vi "FormCalibra9_motorAllON.vi"() -> ()   [LabVIEW 2014]
uses:
  testMachine.ctl
  mainMachine.ctl
  <vilib>/Analysis/baseanly.llb/Mean (DBL).vi
  <vilib>/express/express shared/transition.llb/Dynamic To Waveform Array.vi
  <vilib>/express/express signal manip/GetorSetDDTAttributes/Set DDT Attributes/SetT0.vi
  <vilib>/express/express shared/transition.llb/Waveform Array To Dynamic.vi
  <vilib>/measure/mamon.llb/Trigger Detection for 1 Channel.vi
  <vilib>/express/express signal manip/GetorSetDDTAttributes/Set DDT Attributes/Set DDT Properties.xnode
  <vilib>/Analysis/NI_AALBase.lvlib
  <resource>/objmgr/daqmx.rc
  <vilib>/measure/NI_MAPro.lvlib
panel:
  out "editDistance":dbl caption="Distancia (m)" format="%#_4f"
  in  "Lower level":dbl
  in  "hysteresis":dbl format="%.2p"
  in  "level":dbl format="%.2p"
  out "rpm":bool
  out "deviceName":tag
  out "editTotalWaitLimit":u8
  out "editCountWaitLimit":u8
  out "ledWaitState":bool caption="Wait State"
  out "sliderWaitUpperTime":u8(slide) max=50 scale=0.0..10.0
  out "slideWaitLowerTime":u8(slide) max=30 scale=0.0..1.0
  out "slideWaitTime":u8(slide) scale=0.0..1.0
  out "labelTestTime":string caption="Tempo total de ensaio"
  in  "buttonAcquisition":bool
  in  "editSetWaitTime":u8 caption="Tempo entre ciclos (s)" step=1 format="%0d"
  in  "stop":bool
  out "error out":errorcluster
  out "ledAcquireState":bool caption="Acquire State"
  out "editTotalLowerLimit":u8
  out "editCountLowerLimit":u8
  out "editTotalUpperLimit":u8
  out "editCountUpperLimit":u8
  out "ledEnsaio 3":bool
  out "ledBrakeState":bool caption="Brake State"
  out "ledExitState":bool caption="Exit State"
  out "ledMotorState":bool caption="Motor State"
  out "ledInit2State":bool caption="Init State"
  out "ledBlockState":bool caption="Block State"
  out "ledRunningState":bool caption="Running State"
  out "ledReadyState":bool caption="Ready State"
  out "ledInitState":bool caption="Init State"
  out "mainMachine":T1
  out "testMachine":T2=enum."finish"
  in  "editSetPathToFile":path
  in  "buttonStop":bool
  in  "buttonStart":bool
  out "graphForce":dynamicdata(graph)
  in  "editOffsetForce":dbl caption="Tara" min=0.0 max=100.0 step=0.1
  in  "editSetForce":dbl caption="Fator de conversão"
  out "editForce":dbl caption="Força (Kgf)" format="%#_4f"
  out "graphSpeed":dynamicdata(graph)
  in  "editSetSpeed":dbl caption="Fator de conversão"
  out "editSpeed":dbl caption="Velocidade (km/h)" format="%#_4f"
  out "editEngineSpeed":dbl caption="Rotação (RPM)" format="%#_4f"
  in  "buttonMotor":bool
  in  "buttonBrake":bool
  in  "editSetWaitLowerTime":u8 caption="Tempo de espera (s)"
  in  "editSetWaitUpperTime":u8=3 caption="Tempo de espera (s)"
  in  "editSetNumberOfCycles":u16 caption="Número de ciclos" max=999 step=1 format="%0d"
  in  "editSetLowerLimit":u32 caption="Limite inferior (km/h)"
  in  "editSetUpperLimit":u32 caption="Limite superior (km/h)"
  out "editTempB":dbl caption="Temperatura B (ºC)"
  out "editTempA":dbl caption="Temperatura A (ºC)"
  in  "editSetTempRef":dbl caption="Offset referência" step=0.01 format="%#_2f"
  out "editTempRef":dbl caption="Referência (ºC)"
  out "ledMotor":bool
  out "ledBrake":bool
  out "ledEnsaio":bool
  out "labelTotalCycle":string
  out "labelCurrentCycle":string
  out "labelSystemTitle":string
  in  "editCurrCycleCtr":u32
  in  "velocidade 2":u32
  out "velocidade":u32
  # "Bancada de Frenagem - Ensaio"
  # "Ensaio"
  # "Temperatura"
  # "Rotação"
  # "Célula de Carga"
  # "Configurações do ensaio"
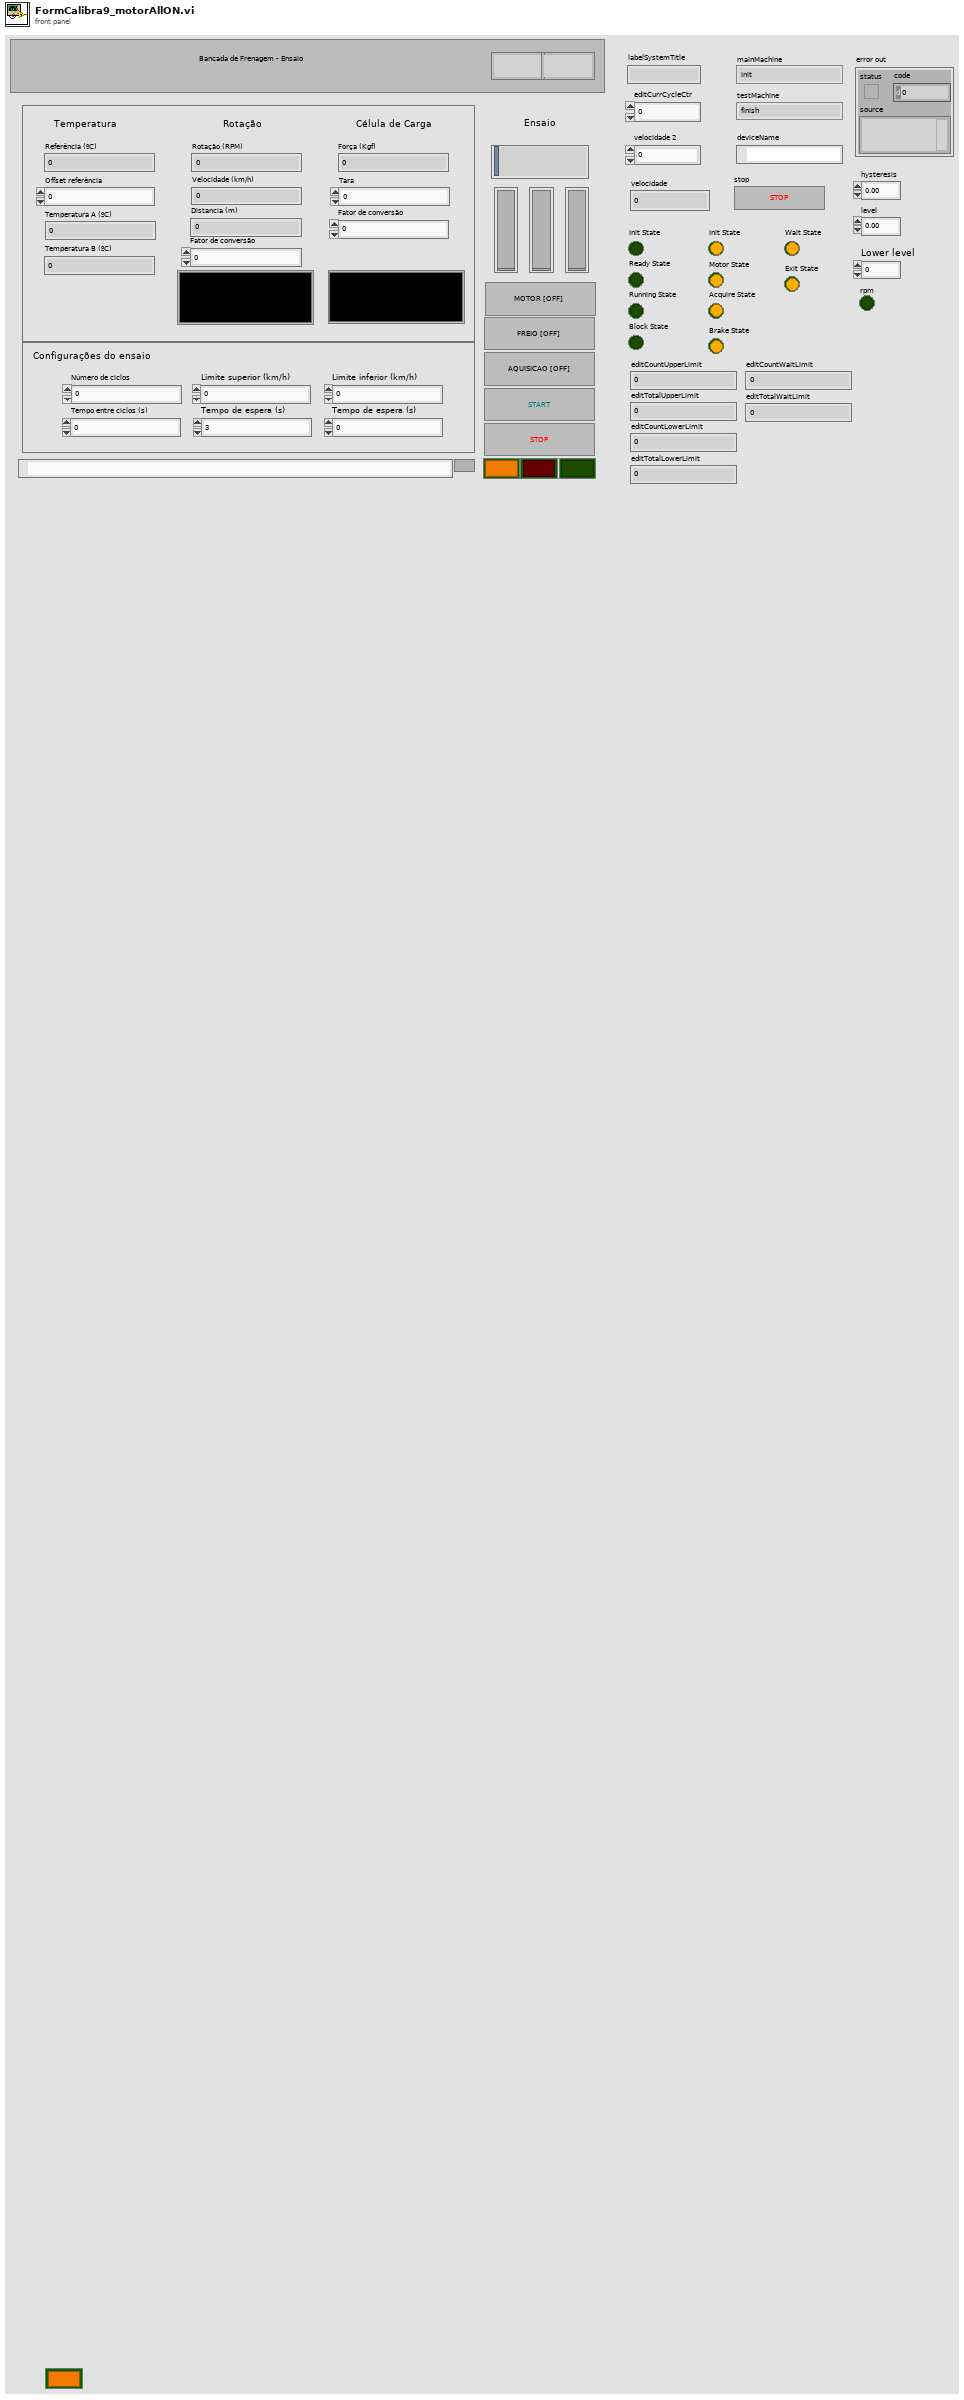
[diagram p1: front panel]
types:
  T1 = typedef "mainMachine.ctl" = enum16{"init", "ready", "running", "blocked", "finish"}
  T2 = typedef "testMachine.ctl" = enum16{"init", "motor", "motor acquire", "brake", "brake acquire", "wait ", "finish", "exit"}
  T3 = enum8{"Enabled", "Disabled", "Disabled and Grayed Out"}
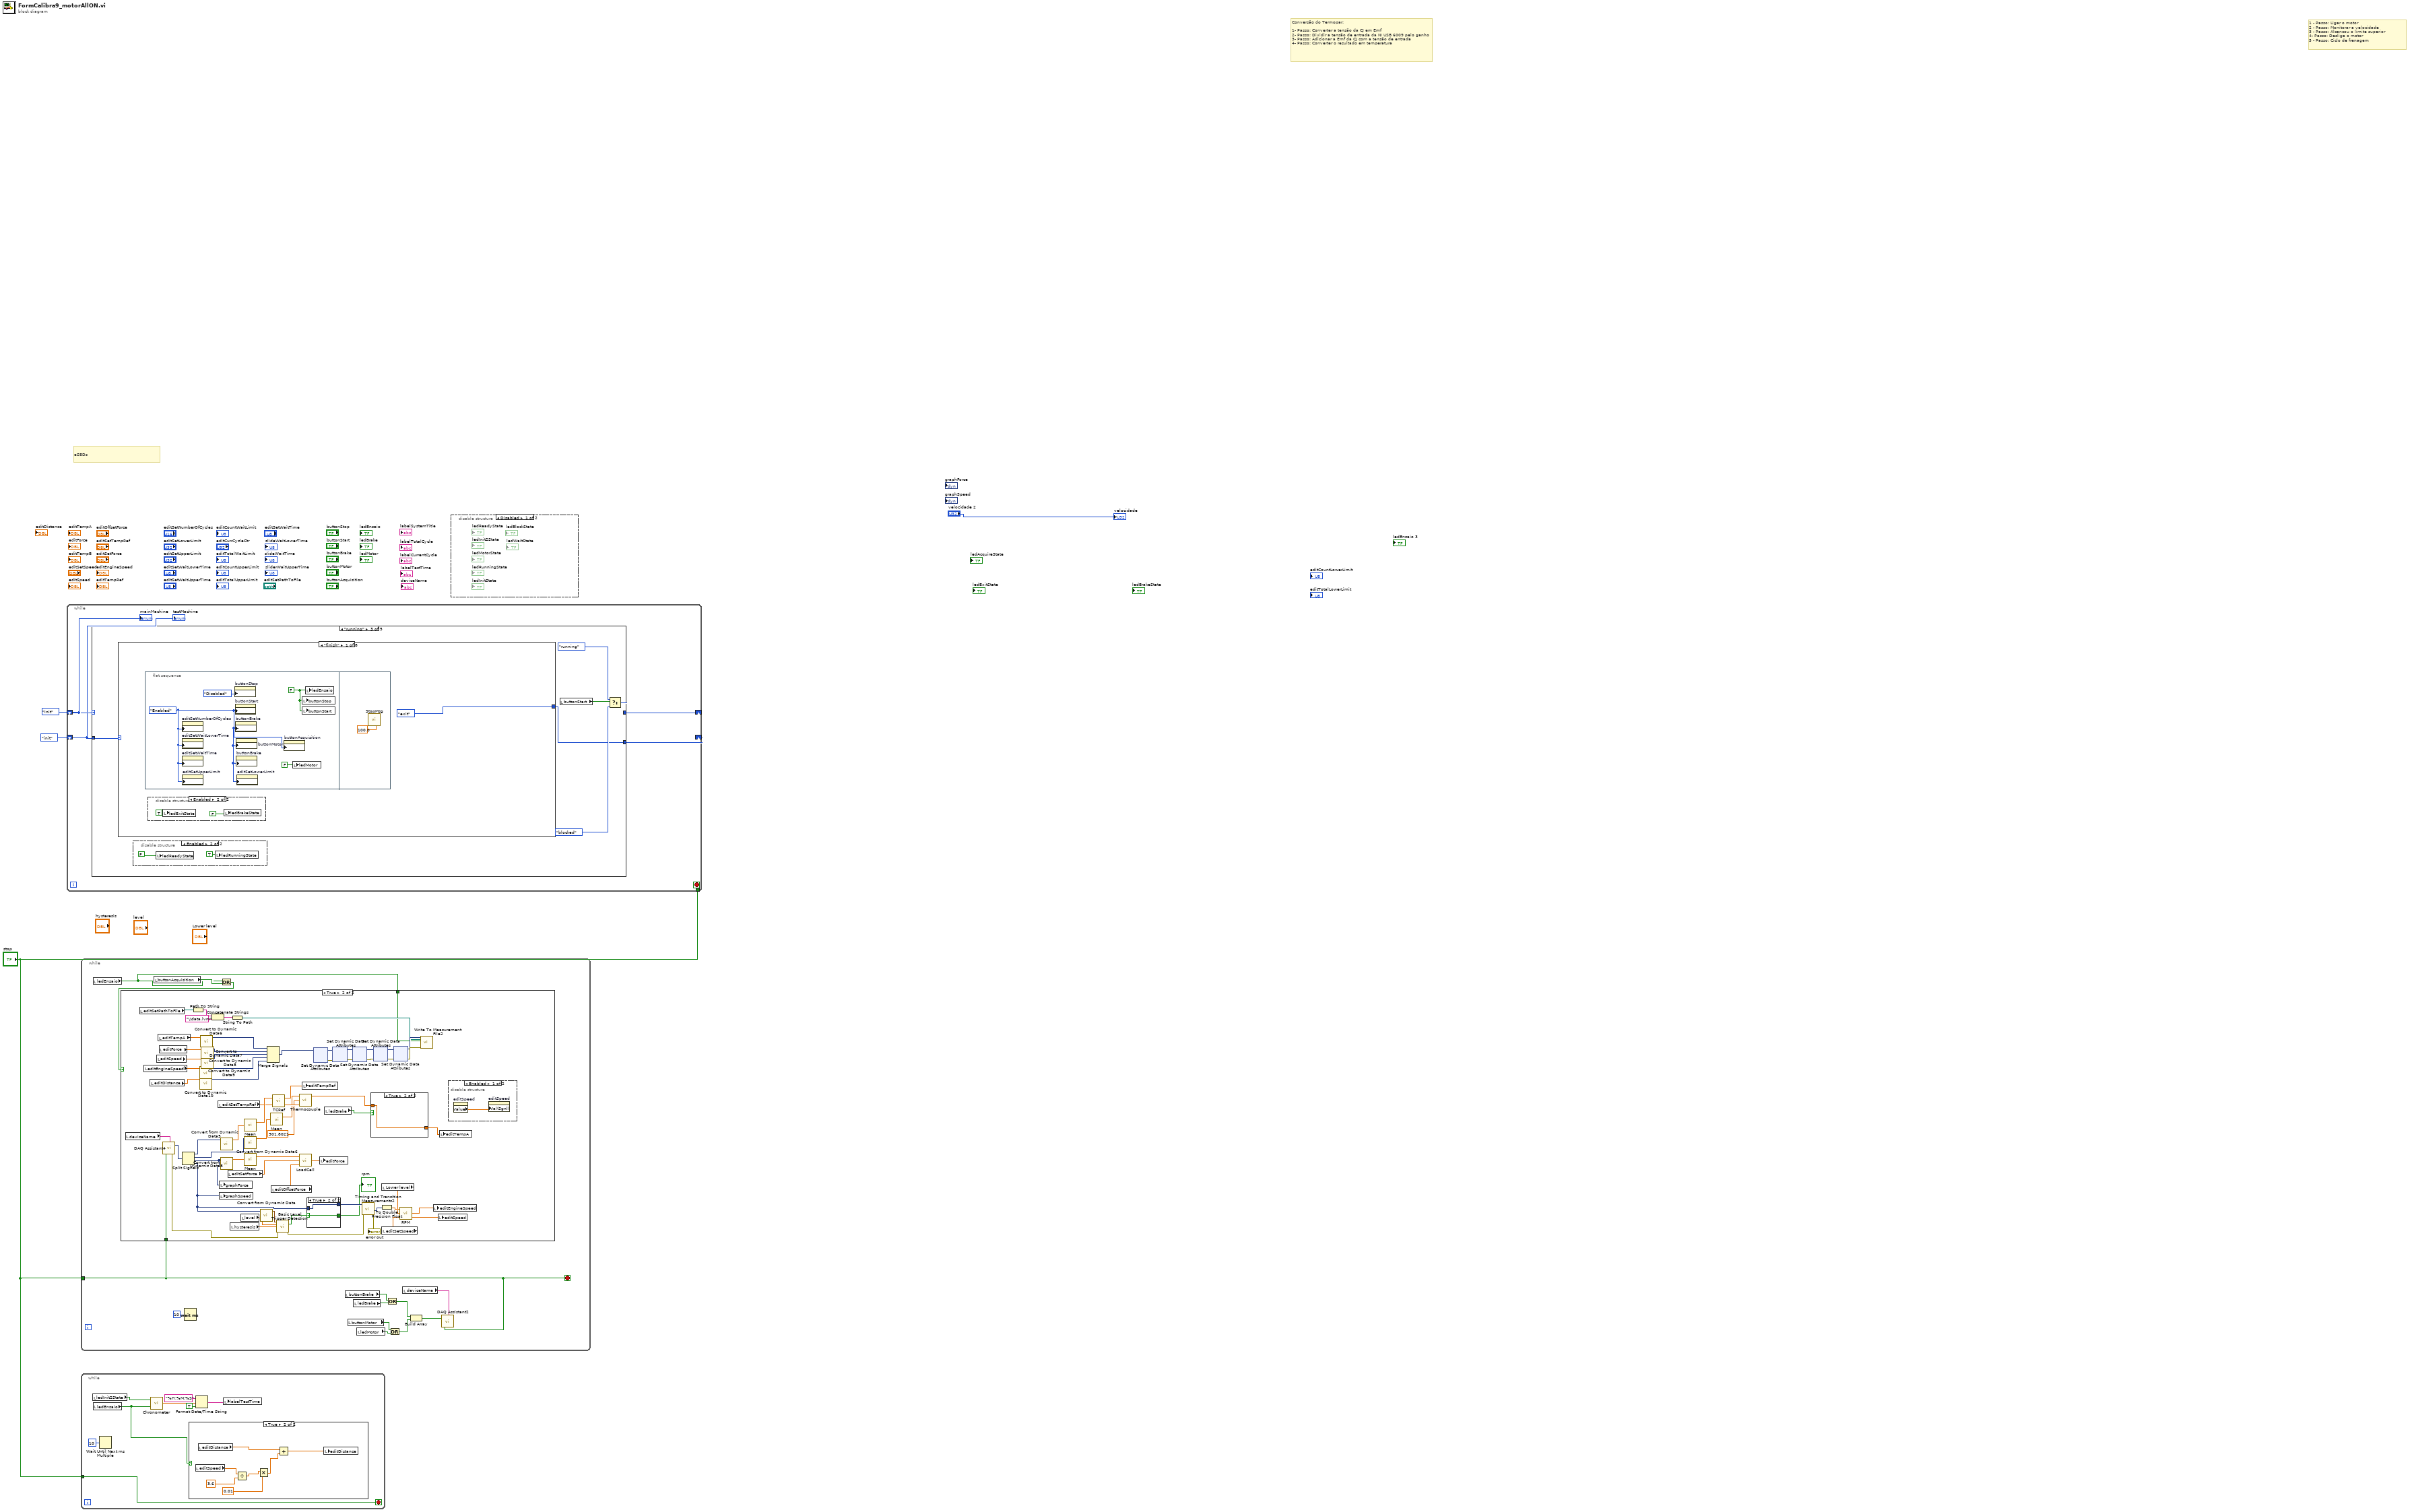
[diagram p0: block diagram]
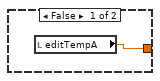
[diagram p5: hidden frame]
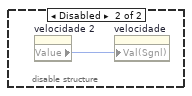
[diagram p7: hidden frame]
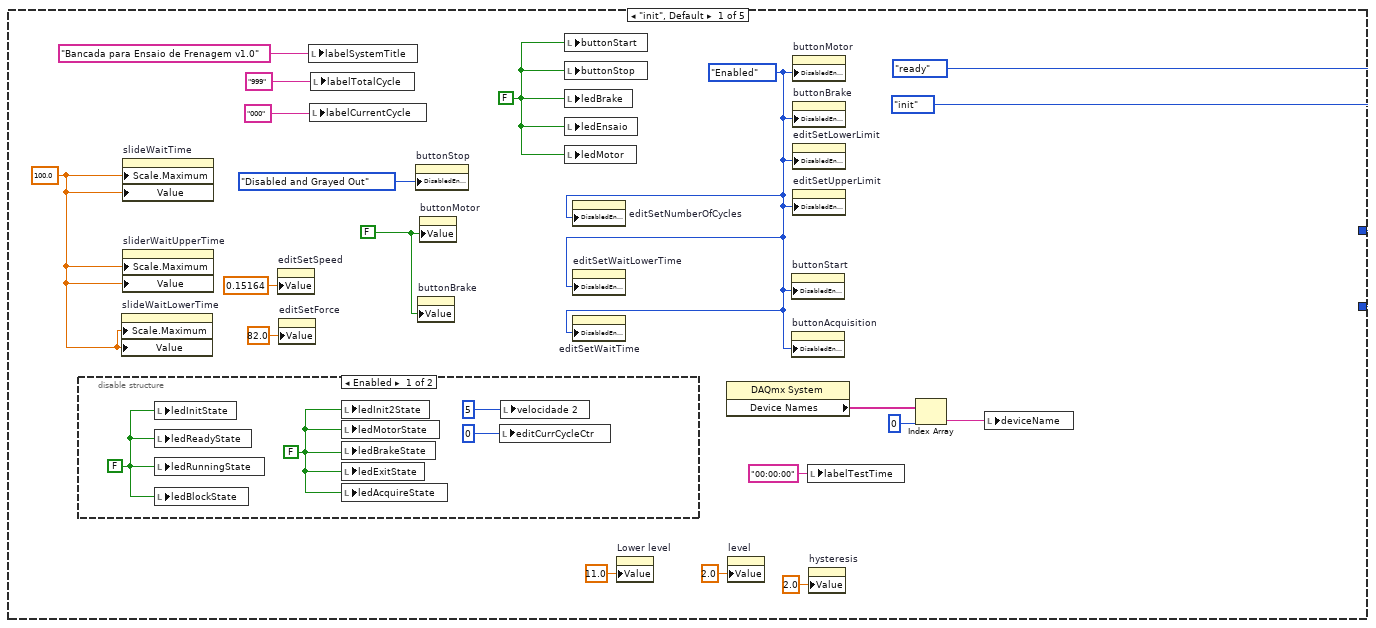
[diagram p8: hidden frame]
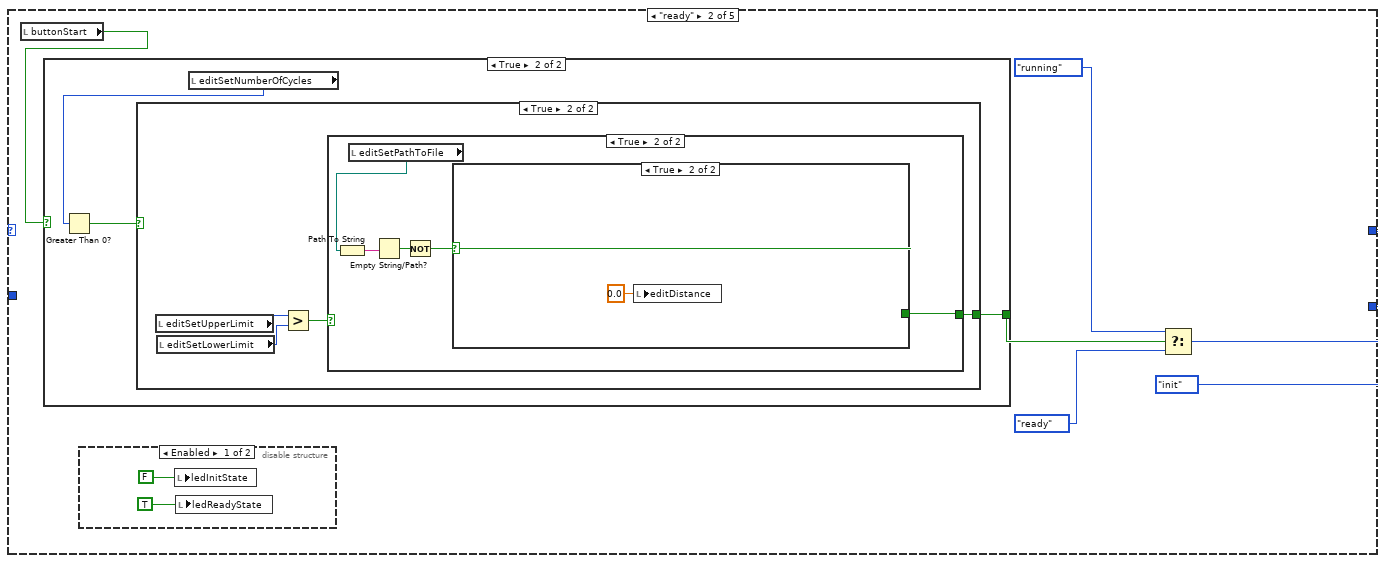
[diagram p10: hidden frame]
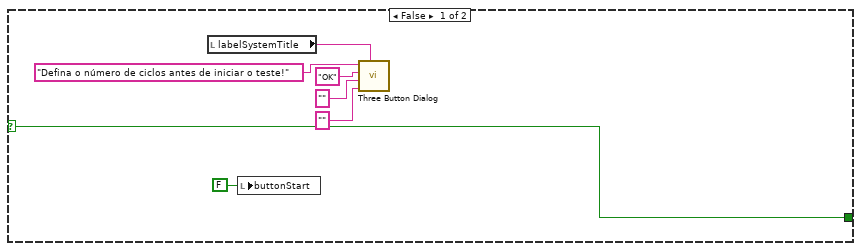
[diagram p13: hidden frame]
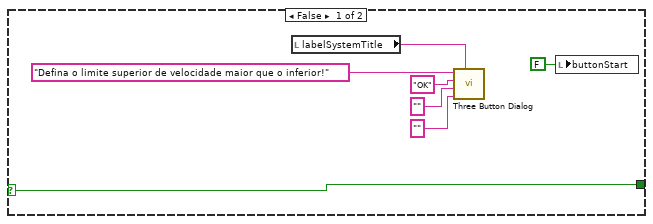
[diagram p14: hidden frame]
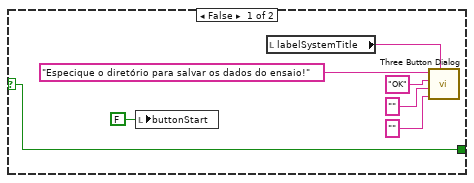
[diagram p15: hidden frame]
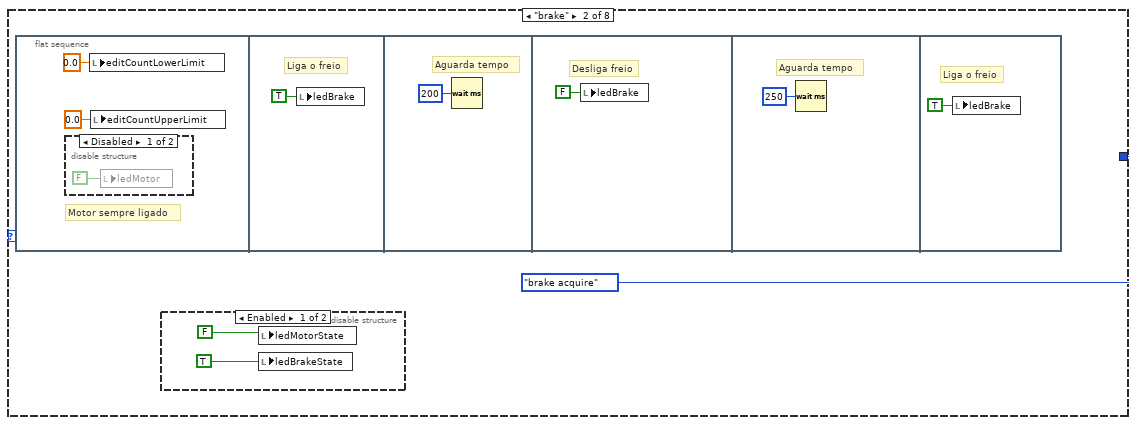
[diagram p18: hidden frame]
diagram:
  # "eSEDs"
  # "1 - Passo: Ligar o motor\n2 - Passo: Monitorar a velocidade\n3 - Passo: Alcancou o limite superior\n4- Passo: Desliga o motor\n5 - Passo: Ciclo de frenagem"
  # "Conversão do Termopar:\n\n1- Passo: Converter a tensão da CJ em Emf\n2- Passo: Dividir a tensão de entrada da NI USB 6009 pelo ganho\n3- Passo: Adicionar a Emf da CJ com a tensão de entrada\n4- Passo: Converter o resultado em temperatura"
  n1 = while {
    shift-right: [w9] -> _
    shift-left: mainMachine."init" ("mainMachine") -> [w6]
    shift-right: [w8] -> _
    shift-left: testMachine."init" ("testMachine") -> [w7]
    tunnel: "stop" -> [w5]
    stop <- w5 stop-if-true
    n2 = case shown="\"running\"" w6 {
      tunnel: [mainMachine."ready" ("mainMachine") w33 w79 w224 mainMachine."finish" ("mainMachine")] -> w9
      tunnel: [testMachine."init" ("testMachine") testMachine."init" ("testMachine") w78 testMachine."init" ("testMachine") testMachine."init" ("testMachine")] -> w8
      tunnel: w7 -> [_ _ w77 _ _]
      frame "init", Default {
        w19 = 100.0 ("Scale.Range:Maximum")
        w20 = T3."Enabled" ("Disabled")
        w21 = FALSE ("buttonMotor")
        w27 = FALSE ("motor")
        n3 = disable-structure shown="Enabled" {
          frame Enabled {
            w29 = FALSE
            w30 = FALSE
            n4 = local write "ledInitState"(w30) -> ()
            n5 = local write "ledReadyState"(w30) -> ()
            n6 = local write "ledRunningState"(w30) -> ()
            n7 = local write "ledBlockState"(w30) -> ()
            n8 = local write "ledInit2State"(w29) -> ()
            n9 = local write "ledMotorState"(w29) -> ()
            n10 = local write "ledBrakeState"(w29) -> ()
            n11 = local write "ledExitState"(w29) -> ()
            n12 = local write "ledAcquireState"(w29) -> ()
            n13 = local write "editCurrCycleCtr"(u32 0 ("currentCycleCtr")) -> ()
            n14 = local write "velocidade 2"(u32 5 ("velocidade 2")) -> ()
          }
          frame Disabled {
          }
        }
        n15 = property on="slideWaitLowerTime" class="Slide (strict)"("Scale.Maximum"=w19, "Value"=w19) -> ()  [unwired: 2 in, 2 out]
        n16 = property on="slideWaitTime" class="Slide (strict)"("Scale.Maximum"=w19, "Value"=w19) -> ()  [unwired: 2 in, 2 out]
        n17 = property on="sliderWaitUpperTime" class="Slide (strict)"("Scale.Maximum"=w19, "Value"=w19) -> ()  [unwired: 2 in, 2 out]
        n18 = property on="editSetSpeed" class="DigNum (strict)"("Value"=0.15164 ("editSetSpeed")) -> ()  [unwired: 2 in, 2 out]
        n19 = property on="editSetForce" class="DigNum (strict)"("Value"=82.0 ("editSetForce")) -> ()  [unwired: 2 in, 2 out]
        n20 = local write "labelSystemTitle"("Bancada para Ensaio de Frenagem v1.0" ("systemTitle")) -> ()
        n21 = local write "labelCurrentCycle"("000" ("currentCycle")) -> ()
        n22 = local write "labelTotalCycle"("999" ("totalCycle")) -> ()
        n23 = property on="buttonStop" class="Bool (strict)"("DisabledEnum"=T3."Disabled and Grayed Out" ("Disabled")) -> ()  [unwired: 2 in, 2 out]
        n24 = property on="buttonBrake" class="Bool (strict)"("Value"=w21) -> ()  [unwired: 2 in, 2 out]
        n25 = property on="buttonMotor" class="Bool (strict)"("Value"=w21) -> ()  [unwired: 2 in, 2 out]
        n26 = local write "buttonStart"(w27) -> ()
        n27 = local write "buttonStop"(w27) -> ()
        n28 = local write "ledBrake"(w27) -> ()
        n29 = local write "ledEnsaio"(w27) -> ()
        n30 = local write "ledMotor"(w27) -> ()
        n31 = property on="editSetNumberOfCycles" class="DigNum (strict)"("DisabledEnum"=w20) -> ()  [unwired: 2 in, 2 out]
        n32 = property on="editSetWaitLowerTime" class="DigNum (strict)"("DisabledEnum"=w20) -> ()  [unwired: 2 in, 2 out]
        n33 = property on="editSetWaitTime" class="DigNum (strict)"("DisabledEnum"=w20) -> ()  [unwired: 2 in, 2 out]
        n34 = property on="Lower level" class="DigNum (strict)"("Value"=11.0 ("Lower level")) -> ()  [unwired: 2 in, 2 out]
        n35 = property class="DAQmx System"() -> ("Device Names"=w18:tag[])  [unwired: 2 in, 2 out]
        n36 = property on="level" class="DigNum (strict)"("Value"=2.0 ("level")) -> ()  [unwired: 2 in, 2 out]
        n37 = property on="buttonStart" class="Bool (strict)"("DisabledEnum"=w20) -> ()  [unwired: 2 in, 2 out]
        n38 = property on="buttonAcquisition" class="Bool (strict)"("DisabledEnum"=w20) -> ()  [unwired: 2 in, 2 out]
        n39 = property on="buttonMotor" class="Bool (strict)"("DisabledEnum"=w20) -> ()  [unwired: 2 in, 2 out]
        n40 = property on="buttonBrake" class="Bool (strict)"("DisabledEnum"=w20) -> ()  [unwired: 2 in, 2 out]
        n41 = property on="editSetLowerLimit" class="DigNum (strict)"("DisabledEnum"=w20) -> ()  [unwired: 2 in, 2 out]
        n42 = property on="editSetUpperLimit" class="DigNum (strict)"("DisabledEnum"=w20) -> ()  [unwired: 2 in, 2 out]
        n43 = local write "labelTestTime"("00:00:00" ("labelTestTime")) -> ()
        n44 = property on="hysteresis" class="DigNum (strict)"("Value"=2.0 ("hysteresis")) -> ()  [unwired: 2 in, 2 out]
        n45 = Index Array(array=w18, index=0) -> (element=w16:tag)
        n46 = local write "deviceName"(w16) -> ()
      }
      frame "ready" {
        n47 = local read "buttonStart"() -> (w36:bool)
        n48 = case shown="True" w36 {
          selector: w36 -> [w41 _]
          tunnel: [w41 w42] -> w35
          frame False {
          }
          frame True {
            n49 = local read "editSetNumberOfCycles"() -> (w43:u16)
            n50 = Greater Than 0?(x=w43) -> (x > 0?=w44:bool)
            n51 = case shown="True" w44 {
              selector: w44 -> [w51 _]
              tunnel: [w51 w52] -> w42
              frame False {
                n52 = local read "labelSystemTitle"() -> (w46:string)
                n53 = local write "buttonStart"(FALSE ("startButton")) -> ()
                n54 = call <vilib>:"Three Button Dialog.vi"("Window Title (\"\")"=w46, "Right Button Text (\"Cancel\")"="" ("Right Button Text (\"Cancel\")"), "Center Button Text (\"No\")"="" ("Center Button Text (\"No\")"), "Left Button Text (\"Yes\")"="OK" ("Left Button Text (\"Yes\")"), "message"="Defina o número de ciclos antes de iniciar o teste!") -> ()  [unwired: 6 in, 1 out]
              }
              frame True {
                n55 = local read "editSetUpperLimit"() -> (w54:u32)
                n56 = local read "editSetLowerLimit"() -> (w53:u32)
                n57 = Greater?(x=w54, y=w53) -> (0:w55:bool)
                n58 = case shown="True" w55 {
                  selector: w55 -> [w62 _]
                  tunnel: [w62 w65] -> w52
                  frame False {
                    n59 = local read "labelSystemTitle"() -> (w57:string)
                    n60 = call <vilib>:"Three Button Dialog.vi"("Window Title (\"\")"=w57, "Right Button Text (\"Cancel\")"="" ("Right Button Text (\"Cancel\")"), "Center Button Text (\"No\")"="" ("Center Button Text (\"No\")"), "Left Button Text (\"Yes\")"="OK" ("Left Button Text (\"Yes\")"), "message"="Defina o limite superior de velocidade maior que o inferior!") -> ()  [unwired: 6 in, 1 out]
                    n61 = local write "buttonStart"(FALSE ("startButton")) -> ()
                  }
                  frame True {
                    n62 = local read "editSetPathToFile"() -> (w67:path)
                    n63 = Path To String(path=w67) -> (string=w66:string)
                    n64 = Empty String/Path?(string/path=w66) -> (empty?=w64:bool)
                    n65 = Not(x=w64) -> (.not. x?=w63:bool)
                    n66 = case shown="True" w63 {
                      selector: w63 -> [w74 w76]
                      tunnel: [w74 w76] -> w65
                      frame False {
                        n67 = local write "buttonStart"(FALSE ("startButton")) -> ()
                        n68 = local read "labelSystemTitle"() -> (w69:string)
                        n69 = call <vilib>:"Three Button Dialog.vi"("Window Title (\"\")"=w69, "Right Button Text (\"Cancel\")"="" ("Right Button Text (\"Cancel\")"), "Center Button Text (\"No\")"="" ("Center Button Text (\"No\")"), "Left Button Text (\"Yes\")"="OK" ("Left Button Text (\"Yes\")"), "message"="Especique o diretório para salvar os dados do ensaio!") -> ()  [unwired: 6 in, 1 out]
                      }
                      frame True {
                        n70 = local write "editDistance"(0.0 ("editDistance")) -> ()
                      }
                    }
                  }
                }
              }
            }
          }
        }
        n71 = disable-structure shown="Enabled" {
          frame Enabled {
            n72 = local write "ledInitState"(FALSE ("ledReady")) -> ()
            n73 = local write "ledReadyState"(TRUE ("ledReady")) -> ()
          }
          frame Disabled {
          }
        }
        n74 = Select(t=mainMachine."running" ("mainMachine"), s=w35, f=mainMachine."ready" ("mainMachine")) -> (s? t:f=w33:T1)
      }
      frame "running" {
        n75 = case shown="\"finish\"" w77 {
          tunnel: [testMachine."exit" ("testMachine") testMachine."brake acquire" ("testMachine") testMachine."motor acquire" ("testMachine") testMachine."motor" ("testMachine") w154 w174 testMachine."exit" ("testMachine") w207] -> w78
          frame "finish" {
            n76 = flat-sequence {
              frame #0 {
                w90 = FALSE ("ledReady")
                w89 = T3."Enabled" ("Disabled")
                n77 = property on="editSetNumberOfCycles" class="DigNum (strict)"("DisabledEnum"=w89) -> ()  [unwired: 2 in, 2 out]
                n78 = property on="editSetWaitLowerTime" class="DigNum (strict)"("DisabledEnum"=w89) -> ()  [unwired: 2 in, 2 out]
                n79 = property on="editSetWaitTime" class="DigNum (strict)"("DisabledEnum"=w89) -> ()  [unwired: 2 in, 2 out]
                n80 = property on="editSetUpperLimit" class="DigNum (strict)"("DisabledEnum"=w89) -> ()  [unwired: 2 in, 2 out]
                n81 = property on="buttonStop" class="Bool (strict)"("DisabledEnum"=T3."Disabled" ("Disabled")) -> ()  [unwired: 2 in, 2 out]
                n82 = property on="buttonStart" class="Bool (strict)"("DisabledEnum"=w89) -> ()  [unwired: 2 in, 2 out]
                n83 = property on="buttonBrake" class="Bool (strict)"("DisabledEnum"=w89) -> ()  [unwired: 2 in, 2 out]
                n84 = property on="buttonMotor" class="Bool (strict)"("DisabledEnum"=w89) -> ()  [unwired: 2 in, 2 out]
                n85 = property on="buttonBrake" class="Bool (strict)"("DisabledEnum"=w89) -> ()  [unwired: 2 in, 2 out]
                n86 = property on="editSetLowerLimit" class="DigNum (strict)"("DisabledEnum"=w89) -> ()  [unwired: 2 in, 2 out]
                n87 = property on="buttonAcquisition" class="Bool (strict)"("DisabledEnum"=w89) -> ()  [unwired: 2 in, 2 out]
                n88 = local write "ledMotor"(FALSE ("motor")) -> ()
                n89 = local write "buttonStop"(w90) -> ()
                n90 = local write "buttonStart"(w90) -> ()
                n91 = local write "ledEnsaio"(w90) -> ()
              }
              frame #1 {
                n92 = call "StopMsg.vi"("Max Value (100)"=100.0) -> ()  [unwired: 8 in, 2 out]
              }
            }
            n93 = disable-structure shown="Enabled" {
              frame Disabled {
              }
              frame Enabled {
                n94 = local write "ledExitState"(TRUE ("ledReady")) -> ()
                n95 = local write "ledBrakeState"(FALSE ("ledReady")) -> ()
              }
            }
          }
          frame "brake" {
            n96 = flat-sequence {
              frame #0 {
                # "Motor sempre ligado"
                n97 = disable-structure shown="Disabled" {
                  frame Disabled {
                    n98 = local write "ledMotor"(FALSE ("motor")) -> ()
                  }
                  frame Enabled {
                  }
                }
                n99 = local write "editCountLowerLimit"(0.0 ("editCountUpperLimit")) -> ()
                n100 = local write "editCountUpperLimit"(0.0 ("editCountUpperLimit")) -> ()
              }
              frame #1 {
                # "Liga o freio"
                n101 = local write "ledBrake"(TRUE ("freio")) -> ()
              }
              frame #2 {
                # "Aguarda tempo"
                n102 = Wait (ms)(milliseconds to wait=u32 200) -> ()  [unwired: 1 out]
              }
              frame #3 {
                # "Desliga freio"
                n103 = local write "ledBrake"(FALSE ("freio")) -> ()
              }
              frame #4 {
                # "Aguarda tempo"
                n104 = Wait (ms)(milliseconds to wait=u32 250) -> ()  [unwired: 1 out]
              }
              frame #5 {
                # "Liga o freio"
                n105 = local write "ledBrake"(TRUE ("freio")) -> ()
              }
            }
            n106 = disable-structure shown="Enabled" {
              frame Enabled {
                n107 = local write "ledMotorState"(FALSE ("ledReady")) -> ()
                n108 = local write "ledBrakeState"(TRUE ("ledReady")) -> ()
              }
              frame Disabled {
              }
            }
          }
          frame "motor" {
            n109 = flat-sequence {
              frame #0 {
                n110 = local read "editCurrCycleCtr"() -> (w109:u32)
                n111 = Increment(x=w109) -> (x+1=w108:u32)
                n112 = local write "editCurrCycleCtr"(w108) -> ()
              }
              frame #1 {
                n113 = local read "editCurrCycleCtr"() -> (w116:u32)
                n114 = local read "editTotalWaitLimit"() -> (w110:u8)
                n115 = local read "editTotalUpperLimit"() -> (w112:u8)
                n116 = local read "editTotalLowerLimit"() -> (w111:u8)
                n117 = local write "editCountLowerLimit"(u8 0 ("editCountLowerLimit")) -> ()
                n118 = local write "editCountWaitLimit"(u8 0 ("editCountWaitLimit")) -> ()
                n119 = local write "editCountUpperLimit"(u8 0 ("editCountUpperLimit")) -> ()
                n120 = Format Into String(format string="%03d", w116) -> (resulting string=w117:string)  [unwired: 2 in, 1 out]
                n121 = property on="sliderWaitUpperTime" class="Slide (strict)"("Value"=w112) -> ()  [unwired: 2 in, 2 out]
                n122 = property on="slideWaitLowerTime" class="Slide (strict)"("Value"=w111) -> ()  [unwired: 2 in, 2 out]
                n123 = property on="slideWaitTime" class="Slide (strict)"("Value"=w110) -> ()  [unwired: 2 in, 2 out]
                n124 = local write "labelCurrentCycle"(w117) -> ()
              }
              frame #2 {
                # "- Liga o motor"
                n125 = local write "ledMotor"(TRUE ("motor")) -> ()
                n126 = property on="buttonStop" class="Bool (strict)"("DisabledEnum"=T3."Enabled" ("Disabled")) -> ()  [unwired: 2 in, 2 out]
                n127 = property on="buttonStart" class="Bool (strict)"("DisabledEnum"=T3."Disabled and Grayed Out" ("Disabled")) -> ()  [unwired: 2 in, 2 out]
              }
            }
            n128 = disable-structure shown="Enabled" {
              frame Enabled {
                n129 = local write "ledInit2State"(FALSE ("ledReady")) -> ()
                n130 = local write "ledBrakeState"(FALSE ("ledReady")) -> ()
                n131 = local write "ledMotorState"(TRUE ("ledReady")) -> ()
              }
              frame Disabled {
              }
            }
          }
          frame "init", Default {
            n132 = stacked-sequence {
              frame #0 {
                w129 = FALSE ("ensaio")
                n133 = property on="buttonBrake" class="Bool (strict)"("Value"=w129) -> ()  [unwired: 2 in, 2 out]
                n134 = local write "ledMotor"(w129) -> ()
                n135 = local write "ledBrake"(w129) -> ()
                n136 = property on="buttonMotor" class="Bool (strict)"("Value"=w129) -> ()  [unwired: 2 in, 2 out]
                n137 = local read "editSetNumberOfCycles"() -> (w136:u16)
                n138 = local read "editSetWaitLowerTime"() -> (w130:u8)
                n139 = local read "editSetWaitUpperTime"() -> (w133:u8)
                n140 = local read "editSetWaitTime"() -> (w124:u8)
                n141 = Multiply(x=w124, y=u32 10) -> (x*y=w125:u32)
                n142 = Multiply(x=w130, y=u32 10) -> (x*y=w128:u32)
                n143 = Format Into String(format string="%03d", w136) -> (resulting string=w137:string)  [unwired: 2 in, 1 out]
                n144 = Multiply(x=w133, y=u32 10) -> (x*y=w127:u32)
                n145 = local write "editTotalLowerLimit"(w128) -> ()
                n146 = local write "editTotalUpperLimit"(w127) -> ()
                n147 = local write "editTotalWaitLimit"(w125) -> ()
                n148 = local write "labelTotalCycle"(w137) -> ()
                n149 = local write "editCurrCycleCtr"(u32 0 ("currentCycleCtr")) -> ()
                n150 = local write "labelCurrentCycle"("000" ("currentCycle")) -> ()
              }
              frame #1 {
                w145 = T3."Disabled" ("Disabled")
                n151 = property on="editSetNumberOfCycles" class="DigNum (strict)"("DisabledEnum"=w145) -> ()  [unwired: 2 in, 2 out]
                n152 = property on="editSetWaitLowerTime" class="DigNum (strict)"("DisabledEnum"=w145) -> ()  [unwired: 2 in, 2 out]
                n153 = property on="editSetWaitTime" class="DigNum (strict)"("DisabledEnum"=w145) -> ()  [unwired: 2 in, 2 out]
                n154 = local read "editTotalUpperLimit"() -> (w148:u8)
                n155 = property on="sliderWaitUpperTime" class="Slide (strict)"("Scale.Maximum"=w148, "Scale.Minimum"=0.0 ("Scale.Range:Minimum"), "Scale.Increment"=1.0 ("Scale.Range:Increment"), "Value"=w148) -> ()  [unwired: 2 in, 2 out]
                n156 = property on="buttonAcquisition" class="Bool (strict)"("DisabledEnum"=w145) -> ()  [unwired: 2 in, 2 out]
                n157 = local read "editTotalLowerLimit"() -> (w142:u8)
                n158 = property on="slideWaitLowerTime" class="Slide (strict)"("Scale.Maximum"=w142, "Scale.Minimum"=0.0 ("Scale.Range:Minimum"), "Scale.Increment"=1.0 ("Scale.Range:Increment"), "Value"=w142) -> ()  [unwired: 2 in, 2 out]
                n159 = local read "editTotalWaitLimit"() -> (w139:u8)
                n160 = property on="slideWaitTime" class="Slide (strict)"("Scale.Maximum"=w139, "Scale.Minimum"=0.0 ("Scale.Range:Minimum"), "Scale.Increment"=1.0 ("Scale.Range:Increment"), "Value"=w139) -> ()  [unwired: 2 in, 2 out]
                n161 = call "StarMsg.vi"("Show"=TRUE, "Max Value (100)"=100.0) -> ()  [unwired: 7 in, 2 out]
                n162 = property on="buttonMotor" class="Bool (strict)"("DisabledEnum"=w145) -> ()  [unwired: 2 in, 2 out]
                n163 = property on="buttonBrake" class="Bool (strict)"("DisabledEnum"=w145) -> ()  [unwired: 2 in, 2 out]
                n164 = property on="editSetLowerLimit" class="DigNum (strict)"("DisabledEnum"=w145) -> ()  [unwired: 2 in, 2 out]
                n165 = property on="editSetUpperLimit" class="DigNum (strict)"("DisabledEnum"=w145) -> ()  [unwired: 2 in, 2 out]
              }
              frame #2 {
                n166 = local write "ledEnsaio"(TRUE ("ensaio")) -> ()
              }
            }
            n167 = disable-structure shown="Enabled" {
              frame Enabled {
                n168 = local write "ledInit2State"(TRUE ("ledReady")) -> ()
              }
              frame Disabled {
              }
            }
          }
          frame "motor acquire" {
            n169 = disable-structure shown="Enabled" {
              frame Enabled {
                n170 = local read "ledAcquireState"() -> (w163:bool)
                n171 = Not(x=w163) -> (.not. x?=w162:bool)
                n172 = local write "ledAcquireState"(w162) -> ()
              }
              frame Disabled {
              }
            }
            n173 = Wait (ms)(milliseconds to wait=u32 100) -> ()  [unwired: 1 out]
            n174 = disable-structure shown="Enabled" {
              disable-tunnel: [w160 w161] -> w153
              frame Enabled {
                n175 = property on="editSpeed" class="DigNum (strict)"() -> ("Value"=w160:dbl)  [unwired: 2 in, 2 out]
              }
              frame Disabled {
                n176 = property on="velocidade" class="DigNum (strict)"() -> ("Value"=w161:u32)  [unwired: 2 in, 2 out]
              }
            }
            n177 = property on="editSetUpperLimit" class="DigNum (strict)"() -> ("Value"=w152:u32)  [unwired: 2 in, 2 out]
            n178 = Greater Or Equal?(x=w153, y=w152) -> (x >= y?=w158:bool)
            n179 = case shown="True" w158 {
              selector: w158 -> [w164 _]
              tunnel: [w164 w165] -> w157
              frame False {
              }
              frame True {
                n180 = flat-sequence {
                  tunnel: [w170] -> w165
                  frame #0 {
                    n181 = local read "editCountUpperLimit"() -> (w168:u8)
                    n182 = Increment(x=w168) -> (x+1=w166:u8)
                    n183 = local write "editCountUpperLimit"(w166) -> ()
                    n184 = local read "editTotalUpperLimit"() -> (w167:u8)
                    n185 = Subtract(x=w167, y=w166) -> (x-y=w169:u8)
                    n186 = property on="sliderWaitUpperTime" class="Slide (strict)"("Value"=w169) -> ()  [unwired: 2 in, 2 out]
                  }
                  frame #1 {
                    n187 = local read "editCountUpperLimit"() -> (w172:u8)
                    n188 = local read "editTotalUpperLimit"() -> (w171:u8)
                    n189 = Greater Or Equal?(x=w172, y=w171) -> (x >= y?=w170:bool)
                  }
                }
              }
            }
            n190 = Select(t=testMachine."brake" ("testMachine"), s=w157, f=testMachine."motor acquire" ("testMachine")) -> (s? t:f=w154:T2)
          }
          frame "brake acquire" {
            n191 = disable-structure shown="Enabled" {
              frame Enabled {
                n192 = local read "ledAcquireState"() -> (w182:bool)
                n193 = Not(x=w182) -> (.not. x?=w181:bool)
                n194 = local write "ledAcquireState"(w181) -> ()
              }
              frame Disabled {
              }
            }
            n195 = Wait (ms)(milliseconds to wait=u32 100) -> ()  [unwired: 1 out]
            n196 = disable-structure shown="Enabled" {
              disable-tunnel: [w183 w184] -> w173
              frame Enabled {
                n197 = property on="editSpeed" class="DigNum (strict)"() -> ("Value"=w183:dbl)  [unwired: 2 in, 2 out]
              }
              frame Disabled {
                n198 = property on="velocidade" class="DigNum (strict)"() -> ("Value"=w184:u32)  [unwired: 2 in, 2 out]
              }
            }
            n199 = property on="editSetLowerLimit" class="DigNum (strict)"() -> ("Value"=w175:u32)  [unwired: 2 in, 2 out]
            n200 = Less Or Equal?(x=w173, y=w175) -> (x <= y?=w179:bool)
            n201 = case shown="True" w179 {
              selector: w179 -> [w185 _]
              tunnel: [w185 w186] -> w177
              frame False {
              }
              frame True {
                n202 = flat-sequence {
                  tunnel: [w192] -> w187
                  tunnel: w187 -> [w196]
                  tunnel: [w195] -> w186
                  frame #0 {
                    n203 = local read "editCountLowerLimit"() -> (w191:u8)
                    n204 = Increment(x=w191) -> (x+1=w190:u8)
                    n205 = local write "editCountLowerLimit"(w190) -> ()
                    n206 = local read "editTotalLowerLimit"() -> (w189:u8)
                    n207 = Subtract(x=w189, y=w190) -> (x-y=w188:u8)
                    n208 = property on="slideWaitLowerTime" class="Slide (strict)"("Value"=w188) -> ()  [unwired: 2 in, 2 out]
                  }
                  frame #1 {
                    n209 = local read "editCountLowerLimit"() -> (w194:u8)
                    n210 = local read "editTotalLowerLimit"() -> (w193:u8)
                    n211 = Greater Or Equal?(x=w194, y=w193) -> (x >= y?=w192:bool)
                  }
                  frame #2 {
                    n212 = case shown="True" w196 {
                      selector: w196 -> [w197 w198]
                      tunnel: [w197 w198] -> w195
                      frame False {
                      }
                      frame True {
                        # "- Desliga o freio"
                        n213 = local write "ledBrake"(FALSE ("freio")) -> ()
                      }
                    }
                  }
                }
              }
            }
            n214 = Select(t=testMachine."wait " ("testMachine"), s=w177, f=testMachine."brake acquire" ("testMachine")) -> (s? t:f=w174:T2)
          }
          frame "exit" {
          }
          frame "wait " {
            # "- Aguarda 0.5s \n- Atualiza o numero de ciclos"
            n215 = flat-sequence {
              tunnel: [w213] -> w201
              frame #0 {
                n216 = local read "editCountWaitLimit"() -> (w209:u8)
                n217 = Increment(x=w209) -> (x+1=w210:u8)
                n218 = local write "editCountWaitLimit"(w210) -> ()
                n219 = local read "editTotalWaitLimit"() -> (w212:u8)
                n220 = Subtract(x=w212, y=w210) -> (x-y=w211:u8)
                n221 = property on="slideWaitTime" class="Slide (strict)"("Value"=w211) -> ()  [unwired: 2 in, 2 out]
              }
              frame #1 {
                n222 = local read "editCountWaitLimit"() -> (w215:u8)
                n223 = local read "editTotalWaitLimit"() -> (w214:u8)
                n224 = Greater Or Equal?(x=w215, y=w214) -> (x >= y?=w213:bool)
              }
            }
            n225 = disable-structure shown="Enabled" {
              frame Enabled {
                n226 = local read "ledWaitState"() -> (w222:bool)
                n227 = Not(x=w222) -> (.not. x?=w221:bool)
                n228 = local write "ledBrakeState"(FALSE ("ledBrakeState")) -> ()
                n229 = local write "ledWaitState"(w221) -> ()
              }
              frame Disabled {
              }
            }
            n230 = Wait (ms)(milliseconds to wait=u32 100) -> ()  [unwired: 1 out]
            n231 = case shown="True" w201 {
              selector: w201 -> [w216 _]
              tunnel: [w216 w220] -> w202
              frame False {
              }
              frame True {
                n232 = local read "editSetNumberOfCycles"() -> (w218:u16)
                n233 = local read "editCurrCycleCtr"() -> (w217:u32)
                n234 = Greater Or Equal?(x=w217, y=w218) -> (x >= y?=w220:bool)
                n235 = Not(x=w220) -> (.not. x?=w219:bool)
                n236 = local write "ledEnsaio"(w219) -> ()
              }
            }
            n237 = Select(t=testMachine."motor" ("testMachine"), s=w201, f=testMachine."wait " ("testMachine")) -> (s? t:f=w203:T2)
            n238 = Select(t=testMachine."finish" ("testMachine"), s=w202, f=w203) -> (s? t:f=w207:T2)
          }
        }
        n239 = disable-structure shown="Enabled" {
          frame Disabled {
          }
          frame Enabled {
            n240 = local write "ledReadyState"(FALSE ("ledReady")) -> ()
            n241 = local write "ledRunningState"(TRUE ("ledReady")) -> ()
          }
        }
        n242 = local read "buttonStart"() -> (w82:bool)
        n243 = Select(t=mainMachine."running" ("mainMachine"), s=w82, f=mainMachine."blocked" ("mainMachine")) -> (s? t:f=w79:T1)
      }
      frame "blocked" {
        n244 = local read "buttonStart"() -> (w228:bool)
        n245 = Select(t=mainMachine."ready" ("mainMachine"), s=w228, f=mainMachine."blocked" ("mainMachine")) -> (s? t:f=w224:T1)
        n246 = local write "ledRunningState"(FALSE ("ledReady")) -> ()
        n247 = local write "ledBlockState"(TRUE ("ledReady")) -> ()
      }
      frame "finish" {
        n248 = local write "ledBlockState"(FALSE ("ledReady")) -> ()
      }
    }
    "mainMachine" <- w6
    "testMachine" <- w7
  }
  n249 = while {
    tunnel: "stop" -> [w241]
    stop <- w241 stop-if-true
    n250 = local read "ledInit2State"() -> (w236:bool)
    n251 = local read "ledEnsaio"() -> (w234:bool)
    n252 = Wait Until Next ms Multiple(millisecond multiple=u32 10) -> ()  [unwired: 1 out]
    n253 = call "Chronometer.vi"("start"=w234, "reset"=w236) -> ("Time"=w240:dbl)
    n254 = case shown="True" w234 {
      frame False {
      }
      frame True {
        n255 = local read "editSpeed"() -> (w246:dbl)
        n256 = local read "editDistance"() -> (w248:dbl)
        n257 = Divide(x=w246, y=3.6) -> (x/y=w244:dbl)
        n258 = Multiply(x=w244, y=0.01) -> (x*y=w243:dbl)
        n259 = Add(x=w248, y=w243) -> (x+y=w242:dbl)
        n260 = local write "editDistance"(w242) -> ()
      }
    }
    n261 = Format Date/Time String(time format string (%c)="%H:%M:%S", seconds (now)=w240, UTC format=TRUE) -> (date/time string=w237:string)
    n262 = local write "labelTestTime"(w237) -> ()
  }
  n263 = while {
    tunnel: "stop" -> [w254]
    stop <- w254 stop-if-true
    n264 = local read "ledEnsaio"() -> (w251:bool)
    n265 = local read "buttonAcquisition"() -> (w253:bool)
    n266 = Wait (ms)(milliseconds to wait=u32 10) -> ()  [unwired: 1 out]
    n267 = Or(x=w251, y=w253) -> (x .or. y?=w252:bool)
    n268 = case shown="True" w252 {
      tunnel: w254 -> [_ w286]
      tunnel: w251 -> [_ w285]
      frame False {
      }
      frame True {
        n269 = local read "deviceName"() -> (w284:tag)
        n270 = local read "editSetPathToFile"() -> (w306:path)
        n271 = local read "editEngineSpeed"() -> (w268:dbl)
        n272 = local read "editDistance"() -> (w269:dbl)
        n273 = local read "editSpeed"() -> (w266:dbl)
        n274 = local read "editTempA"() -> (w318:dbl)
        n275 = local read "editForce"() -> (w267:dbl)
        n276 = call "DAQ Assistant4"("stop (F)"=w286, "device name"=w284) -> ("data"=w288:dynamicdata, "error out"=w283:errorcluster)  [unwired: 14 in, 2 out]
        n277 = Split Signals(w288) -> (w265:dynamicdata, w264:dynamicdata, w263:dynamicdata, w262:dynamicdata)  [unwired: 4 in]
        n278 = Path To String(path=w306) -> (string=w305:string)
        n279 = call "Convert to Dynamic Data9"("Double"=w268) -> ("Dynamic Data Type"=w322:dynamicdata)  [unwired: 3 in]
        n280 = call "Convert to Dynamic Data10"("Double"=w269) -> ("Dynamic Data Type"=w323:dynamicdata)  [unwired: 3 in]
        n281 = call "Convert to Dynamic Data6"("Double"=w318) -> ("Dynamic Data Type"=w319:dynamicdata)  [unwired: 3 in]
        n282 = call "Convert to Dynamic Data7"("Double"=w267) -> ("Dynamic Data Type"=w320:dynamicdata)  [unwired: 3 in]
        n283 = call "Convert to Dynamic Data8"("Double"=w266) -> ("Dynamic Data Type"=w321:dynamicdata)  [unwired: 3 in]
        n284 = Concatenate Strings(w305, "\\data.lvm" ("string")) -> (w308:string)
        n285 = local read "editSetTempRef"() -> (w290:dbl)
        n286 = local write "graphForce"(w263) -> ()
        n287 = local write "graphSpeed"(w262) -> ()
        n288 = call "Convert from Dynamic Data5"("Dynamic Data Type"=w265) -> ("Array"=w303:dbl[])  [unwired: 3 in]
        n289 = call "Convert from Dynamic Data8"("Dynamic Data Type"=w263) -> ("Array"=w292:dbl[])  [unwired: 3 in]
        n290 = local read "editSetForce"() -> (w301:dbl)
        n291 = local read "hysteresis"() -> (w275:dbl)
        n292 = String To Path(string=w308) -> (path=w309:path)
        n293 = local read "level"() -> (w274:dbl)
        n294 = call-poly <vilib>:"Mean.vi"("X"=w303) -> ("mean"=w304:dbl)  [unwired: 1 out]
        n295 = call "Convert from Dynamic Data6"("Dynamic Data Type"=w264) -> ("Array"=w291:dbl[])  [unwired: 3 in]
        n296 = call-poly <vilib>:"Mean.vi"("X"=w292) -> ("mean"=w296:dbl)  [unwired: 1 out]
        n297 = call "Convert from Dynamic Data"("Dynamic Data Type"=w262) -> ("Waveform"=w280:waveform(dbl))  [unwired: 3 in]
        n298 = Merge Signals(w319, w320, w321, w322, w323) -> (w324:dynamicdata)
        n299 = call-poly <vilib>:"Mean.vi"("X"=w291) -> ("mean"=w293:dbl)  [unwired: 1 out]
        n300 = local read "editOffsetForce"() -> (w302:dbl)
        n301 = call "TCRef.vi"("offset"=w290, "data"=w304) -> ("emf(mV)"=w295:dbl, "temp (degC)"=w289:dbl)
        n302 = call-poly <vilib>:"Basic Level Trigger Detection.vi"("signal in"=w280, "level"=w274, "hysteresis"=w275, "error in (no error)"=w283) -> ("trigger detected?"=w279:bool, "error out"=w282:errorcluster)  [unwired: 9 in, 1 out]
        n303 = call "Thermocouple.vi"("cj(mV)"=w295, "factor"=301.8021, "data"=w293) -> ("temp(degC)"=w271:dbl)  [unwired: 2 out]
        n304 = call "LoadCell.vi"("tara"=w302, "factor"=w301, "data"=w296) -> ("force (Kgf)"=w298:dbl)
        n305 = local write "editTempRef"(w289) -> ()
        n306 = case shown="True" w279 {
          selector: w279 -> [w329 w330]
          tunnel: w262 -> [_ w331]
          tunnel: [_ w331] -> w281
          tunnel: [w329 w330] -> w278
          frame False {
          }
          frame True {
          }
        }
        "rpm" <- w278
        n307 = xnode ("Set Dynamic Data Attributes")("Signals In"=w324) -> ("Signals Out"=w310:dynamicdata, "error out"=w312:errorcluster)  [unwired: 4 in]
        n308 = local write "editForce"(w298) -> ()
        n309 = local read "ledBrake"() -> (w272:bool)
        n310 = xnode ("Set Dynamic Data Attributes")("Signals In"=w310, "error in"=w312) -> ("Signals Out"=w311:dynamicdata, "error out"=w313:errorcluster)  [unwired: 3 in]
        n311 = xnode ("Set Dynamic Data Attributes")("Signals In"=w311, "error in"=w313) -> ("Signals Out"=w325:dynamicdata, "error out"=w314:errorcluster)  [unwired: 3 in]
        n312 = call "Timing and Transition Measurements2"("error in (no error)"=w282, "Signals"=w281) -> ("error out"=→"error out":errorcluster, "Frequency"=w277:dynamicdata)  [unwired: 8 in]
        n313 = case shown="True" w272 {
          tunnel: w271 -> [_ w328]
          tunnel: [w327 w328] -> w270
          frame False {
            n314 = local read "editTempA"() -> (w327:dbl)
          }
          frame True {
          }
        }
        n315 = xnode ("Set Dynamic Data Attributes")("Signals In"=w325, "error in"=w314) -> ("Signals Out"=w326:dynamicdata, "error out"=w315:errorcluster)  [unwired: 3 in]
        n316 = To Double Precision Float(number=w277) -> (double precision float=w276:dbl)
        n317 = local read "Lower level"() -> (w273:dbl)
        n318 = local read "editSetSpeed"() -> (w297:dbl)
        n319 = xnode ("Set Dynamic Data Attributes")("Signals In"=w326, "error in"=w315) -> ("Signals Out"=w316:dynamicdata, "error out"=w317:errorcluster)  [unwired: 3 in]
        n320 = call "RPM.vi"("factor"=w297, "Lower level"=w273, "data"=w276) -> ("km/h"=w300:dbl, "RPM"=w299:dbl)  [unwired: 1 out]
        n321 = call "Write To Measurement File2"("Signals"=w316, "Enable"=w285, "error in (no error)"=w317, "Filename"=w309) -> ()  [unwired: 13 in, 3 out]
        n322 = local write "editEngineSpeed"(w299) -> ()
        n323 = local write "editSpeed"(w300) -> ()
        n324 = local write "editTempA"(w270) -> ()
        n325 = disable-structure shown="Enabled" {
          frame Enabled {
            n326 = property on="editSpeed" class="DigNum (strict)"() -> ("Value"=w332:dbl)  [unwired: 2 in, 2 out]
            n327 = property on="editSpeed" class="DigNum (strict)"("Val(Sgnl)"=w332) -> ()  [unwired: 2 in, 2 out]
          }
          frame Disabled {
            n328 = property on="velocidade 2" class="DigNum (strict)"() -> ("Value"=w333:u32)  [unwired: 2 in, 2 out]
            n329 = property on="velocidade" class="DigNum (strict)"("Val(Sgnl)"=w333) -> ()  [unwired: 2 in, 2 out]
          }
        }
      }
    }
    n330 = local read "buttonBrake"() -> (w258:bool)
    n331 = local read "buttonMotor"() -> (w256:bool)
    n332 = local read "ledBrake"() -> (w260:bool)
    n333 = local read "ledMotor"() -> (w257:bool)
    n334 = Or(x=w258, y=w260) -> (x .or. y?=w259:bool)
    n335 = Or(x=w256, y=w257) -> (x .or. y?=w255:bool)
    n336 = local read "deviceName"() -> (w249:tag)
    n337 = Build Array(w259, w255) -> (w261:bool[])
    n338 = call "DAQ Assistant2"("data"=w261, "stop (T)"=w254, "device name"=w249) -> ()  [unwired: 15 in, 2 out]
  }
  n339 = disable-structure shown="Disabled" {
    frame Disabled {
    }
    frame Enabled {
    }
  }
  "velocidade" <- "velocidade 2"
